vi "CargoStateControl.vi"(9 "Elevator State":string="Cargo_Feeder") -> ()   [LabVIEW 2018]
uses:
  RobotStates.vi
  Inputs_DriverStation.vi
  SensorReadings.vi
panel:
  in  "Threshold (ms)":u32=300
  out "Intake Velocity":dbl
  in  "Current Threshold (A)":dbl=15.0
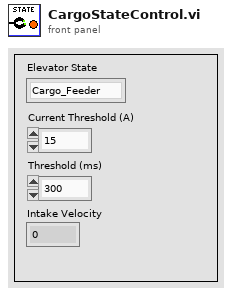
[diagram p1: front panel]
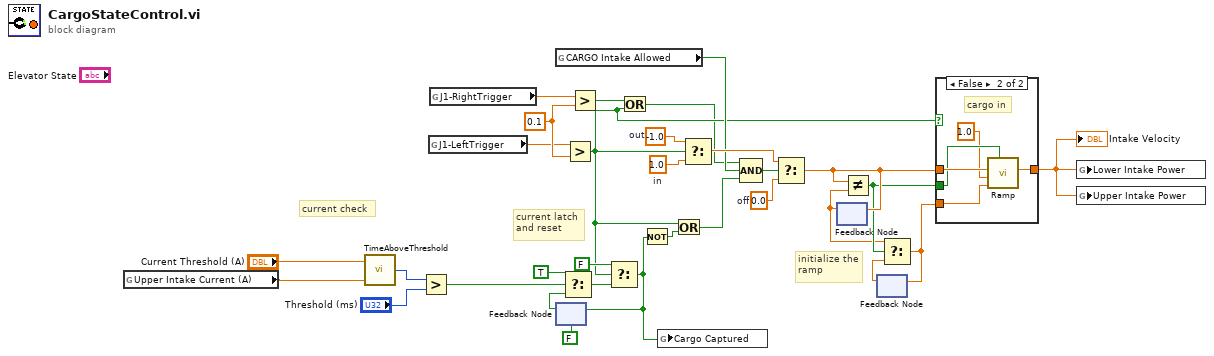
[diagram p0: block diagram]
diagram:
  w9 = 0.1 ("y")
  w28 = 0.0  # off
  w29 = 1.0  # in
  w30 = -1.0  # out
  # "initialize the\nramp"
  # "current latch\nand reset"
  # "current check"
  n1 = global read "SensorReadings.vi" "Upper Intake Current (A)"() -> (w1:dbl)
  n2 = call "TimeAboveThreshold.vi"("Current Value"=w1, "Threshold"="Current Threshold (A)") -> ("Time Above"=w26:u32)  [unwired: 3 in]
  n3 = Greater?(x=w26, y="Threshold (ms)") -> (0:w23:bool)
  n4 = global read "Inputs_DriverStation.vi" "J1-LeftTrigger"() -> (w3:dbl)
  n5 = global read "Inputs_DriverStation.vi" "J1-RightTrigger"() -> (w4:dbl)
  n6 = global read "RobotStates.vi" "CARGO Intake Allowed"() -> (w10:bool)
  n7 = feedback #1(FALSE) -> (w20:bool)
  n8 = Select(t=TRUE, s=w23, f=w20) -> (s? t:f=w19:bool)
  n9 = Greater?(x=w3, y=w9) -> (0:w8:bool)
  n10 = Greater?(x=w4, y=w9) -> (0:w7:bool)
  n11 = Select(t=FALSE, s=w8, f=w19) -> (s? t:f=w2:bool)
  n12 = feedback-in #1(w2) -> ()
  n13 = Or(x=w7, y=w8) -> (x .or. y?=w5:bool)
  n14 = Not(x=w2) -> (.not. x?=w24:bool)
  n15 = global write "SensorReadings.vi" "Cargo Captured"(w2) -> ()
  n16 = Or(x=w8, y=w24) -> (x .or. y?=w11:bool)
  n17 = Select(t=w30, s=w8, f=w29) -> (s? t:f=w31:dbl)
  n18 = Compound Arithmetic op=AND(w5, w10, w11) -> (w12:bool)
  n19 = Select(t=w31, s=w12, f=w28) -> (s? t:f=w17:dbl)
  n20 = feedback-in #2(w17) -> ()
  n21 = feedback #2() -> (w15:dbl)  [unwired: 1 in]
  n22 = Not Equal?(x=w17, y=w15) -> (x != y?=w16:bool)
  n23 = feedback #3() -> (w13:dbl)  [unwired: 1 in]
  n24 = Select(t=w15, s=w16, f=w13) -> (s? t:f=w14:dbl)
  n25 = feedback-in #3(w14) -> ()
  n26 = case shown="False" w8 {
    tunnel: [w32 w36] -> w6
    tunnel: w17 -> [w32 w37]
    tunnel: w16 -> [_ w35]
    tunnel: w14 -> [_ w34]
    frame True {
      # "cargo out"
    }
    frame False {
      # "cargo in"
      n27 = call "Ramp.vi"("Target Value"=w37, "Ramp Time"=1.0, "Inital Value"=w34, "reint"=w35) -> ("Ramped  Value"=w36:dbl)  [unwired: 6 in]
    }
  }
  "Intake Velocity" <- w6
  n28 = global write "RobotStates.vi" "Lower Intake Power"(w6) -> ()
  n29 = global write "RobotStates.vi" "Upper Intake Power"(w6) -> ()
